vi "ABAPI Dist Does File Exist.vi"(4 "error in (no error)":errorcluster, 7 "path":path) -> (0 "error out":errorcluster, 2 "exists?":bool, 3 "dup path":path)   [LabVIEW 2020]
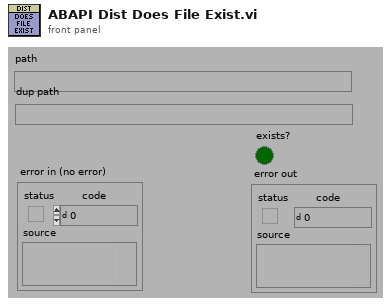
[diagram p1: front panel]
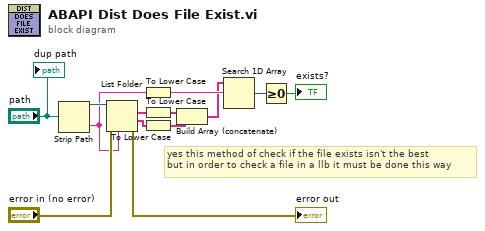
[diagram p0: block diagram]
diagram:
  # "yes this method of check if the file exists isn't the best\nbut in order to check a file in a llb it must be done this way"
  n1 = Strip Path(path="path") -> (stripped path=w13:path, name=w1:string)
  n2 = List Folder(path=w13, pattern=w1, error in="error in (no error)") -> (filenames=w11:string[], folder names=w9:string[], error out=→"error out":errorcluster)  [unwired: 1 in, 1 out]
  n3 = To Lower Case(string=w1) -> (all lower case string=w10:string)
  n4 = To Lower Case(string=w11) -> (all lower case string=w8:string[])
  n5 = To Lower Case(string=w9) -> (all lower case string=w3:string[])
  n6 = Build Array (concatenate)(w8, w3) -> (w7:string[])
  n7 = Search 1D Array(1D array=w7, element=w10) -> (index of element=w6:i32)  [unwired: 1 in]
  n8 = Greater Or Equal To 0?(x=w6) -> (x >= 0?=→"exists?":bool)
  "dup path" <- "path"
